vi "Make.vi"(8 "error in (no error)":errorcluster, 11 "Electrical in":refnum<class "Petrol.lvclass">) -> (0 "error out":errorcluster, 3 "Electrical out":refnum<class "Petrol.lvclass">)   [LabVIEW 2014, in "Petrol.lvclass"]
uses:
  Petrol.lvclass
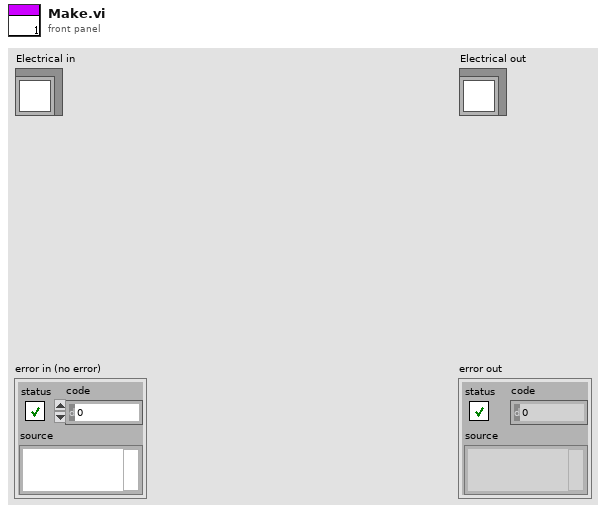
[diagram p1: front panel]
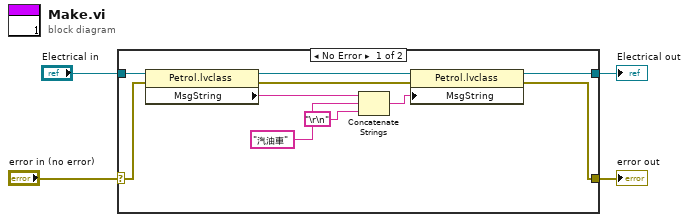
[diagram p0: block diagram]
diagram:
  n1 = case shown="No Error" "error in (no error)" {
    selector: "error in (no error)" -> [w14 w16]
    tunnel: [w11 w16] -> w4
    tunnel: [w9 w15] -> w3
    tunnel: "Electrical in" -> [w12 w15]
    frame No Error {
      n2 = property class="Petrol.lvclass"(reference=w12, error in=w14) -> (reference out=w10:refnum<class "Petrol.lvclass">, error out=w13:errorcluster, "MsgString"=w8:string)
      n3 = Concatenate Strings(w8, "汽油車", "\r\n") -> (w7:string)
      n4 = property class="Petrol.lvclass"(reference=w10, error in=w13, "MsgString"=w7) -> (reference out=w9:refnum<class "Petrol.lvclass">, error out=w11:errorcluster)
    }
    frame Error {
    }
  }
  "error out" <- w4
  "Electrical out" <- w3
